vi "Convert Dialog Options to Variant.vi"(8 "error in (no error)":errorcluster, 11 "dialog options":T1={"angle mode"=1, "picture pixels per unit"=30.0, "close window on exit"=FALSE, "window behavior"=enum."Default"} {"angle mode" items=["Degrees", "Radians"]}) -> (0 "error out":errorcluster, 3 "dialog options variant":variant)   [LabVIEW 2017, in "NI_Robotics_Configure Steering Frame.lvlib"]
uses:
  <vilib>/robotics/Dialog/Configure Steering Frame/NI_Robotics_Configure Steering Frame.lvlib
  <vilib>/robotics/Dialog/Configure Steering Frame/Dialog Options.ctl
  <vilib>/robotics/Dialog/Configure Steering Frame/Angle Mode.ctl
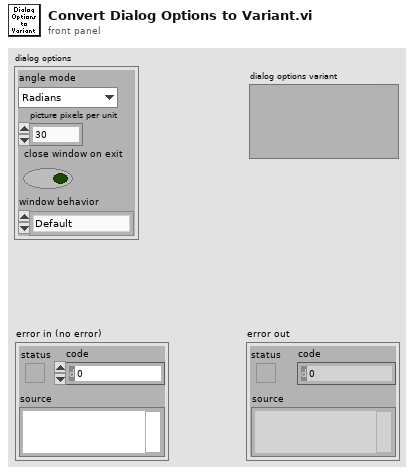
[diagram p1: front panel]
types:
  T1 = typedef "NI_Robotics_Configure Steering Frame.lvlib/Dialog Options.ctl" = cluster{"angle mode":T2, "picture pixels per unit":dbl, "close window on exit":bool, "window behavior":enum32{"Invalid", "Default", "Floating", "Floating/Auto-Hide", "Modal"}}
  T2 = typedef "NI_Robotics_Configure Steering Frame.lvlib/Angle Mode.ctl" = u16
  T3 = enum32{"Invalid", "Default", "Floating", "Floating/Auto-Hide", "Modal"}
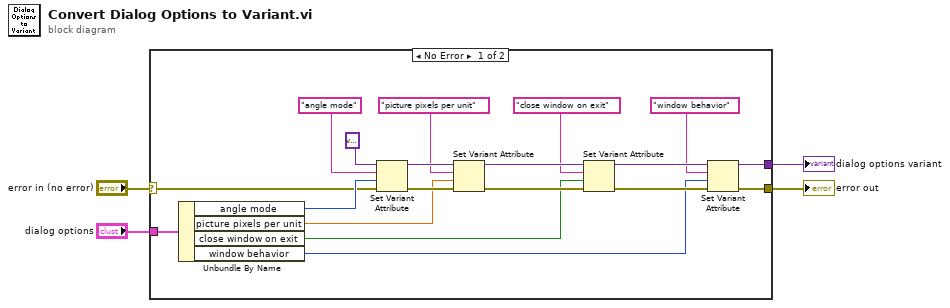
[diagram p0: block diagram]
diagram:
  n1 = case shown="No Error" "error in (no error)" {
    selector: "error in (no error)" -> [w6 w24]
    tunnel: "dialog options" -> [w23 _]
    tunnel: [w7 w24] -> w3
    tunnel: [w5 _] -> w1
    frame No Error {
      n2 = Unbundle By Name(w23) -> ("angle mode"=w20:T2, "picture pixels per unit"=w16:dbl, "close window on exit"=w12:bool, "window behavior"=w8:T3)
      n3 = Set Variant Attribute(Variant=variant ("variant"), name="angle mode", value=w20, error in=w6) -> (Variant out=w19:variant, error out=w18:errorcluster)  [unwired: 1 out]
      n4 = Set Variant Attribute(Variant=w19, name="picture pixels per unit", value=w16, error in=w18) -> (Variant out=w15:variant, error out=w14:errorcluster)  [unwired: 1 out]
      n5 = Set Variant Attribute(Variant=w15, name="close window on exit", value=w12, error in=w14) -> (Variant out=w11:variant, error out=w10:errorcluster)  [unwired: 1 out]
      n6 = Set Variant Attribute(Variant=w11, name="window behavior", value=w8, error in=w10) -> (Variant out=w5:variant, error out=w7:errorcluster)  [unwired: 1 out]
    }
    frame Error {
    }
  }
  "error out" <- w3
  "dialog options variant" <- w1
